vi "C2_controltower.vi"() -> ()   [LabVIEW 2012]
uses:
  <vilib>/LabVIEW Targets/FPGA/cRIO/cRIO-9505/controls.llb/_nicrio_cRIO-9505_DriveStatus.ctl
  <vilib>/FPGAPlugInAG/cRIO-9074/niLvFpga_Open_cRIO-9074.vi
  <vilib>/Utility/error.llb/Error Cluster From Error Code.vi
  <vilib>/rvi/errors/niLvFpgaAdjustHostInterfaceError.vi
  <vilib>/FPGAPlugInAG/cRIO-9074/niLvFpga_Close_cRIO-9074.vi
  <vilib>/rvi/interface/nirviOpenFPGA/nirviOpenFPGA.xnode
  FPGA Bitfiles/bbauvsbRIO_FPGATarget_FPGA9505Thruster_WhZwZzeic1g.lvbitx
  <vilib>/rvi/interface/nirviReadWriteControl/nirviReadWriteControl.xnode
  <vilib>/rvi/interface/nirviCloseFPGA/nirviCloseFPGA.xnode
  NiFpgaLv.dll
  <instrlib>/Ocean Server OS4000/Ocean Server OS4000.lvlib
panel:
  in  "Roll PID Gains":T1={"proportional gain (Kc)"=1.0, "integral time (Ti, min)"=0.01, "derivative time (Td, min)"=0.0}
  in  "Roll Setpoint":dbl
  out "Pwm Output":dbl
  out "Actual Roll":dbl
  out "Actual Heading":dbl
  in  "Baud Rate":u32(ring)=19200
  in  "Reset (True)":bool=TRUE
  in  "ID Query (False)":bool
  in  "Heading PID Gains":T1={"proportional gain (Kc)"=1.0, "integral time (Ti, min)"=0.01, "derivative time (Td, min)"=0.0}
  in  "Heading Setpoint":dbl
  out "Pwm Output":dbl
  in  "Manual Surge":dbl(slide)
  in  "Manual Yaw":dbl(slide)
  in  "Manual Depth":dbl(slide)
  in  "Manual Roll":dbl(slide)
  in  "Control Mode":T2(ring)
  in  "Depth PID Gains":T1={"proportional gain (Kc)"=1.0, "integral time (Ti, min)"=0.01, "derivative time (Td, min)"=0.0}
  in  "Depth Setpoint":dbl
  out "Pwm Output":dbl
  out "Actual Depth (m)":dbl(slide)
  in  "Atm Offset":dbl
  out "PSI":dbl(knob)
  out "Current Sense 2":i16
  out "Current Sense 1":i16
  out "Drive Status 1":T3
  out "Drive Status 2":T3
  in  "Enable 2":bool
  in  "Enable 1":bool
  in  "Disable 2":bool
  in  "Disable 1":bool
  in  "resource name":tag="RIO0::INSTR"
  out "error out":errorcluster
  in  "stop":bool
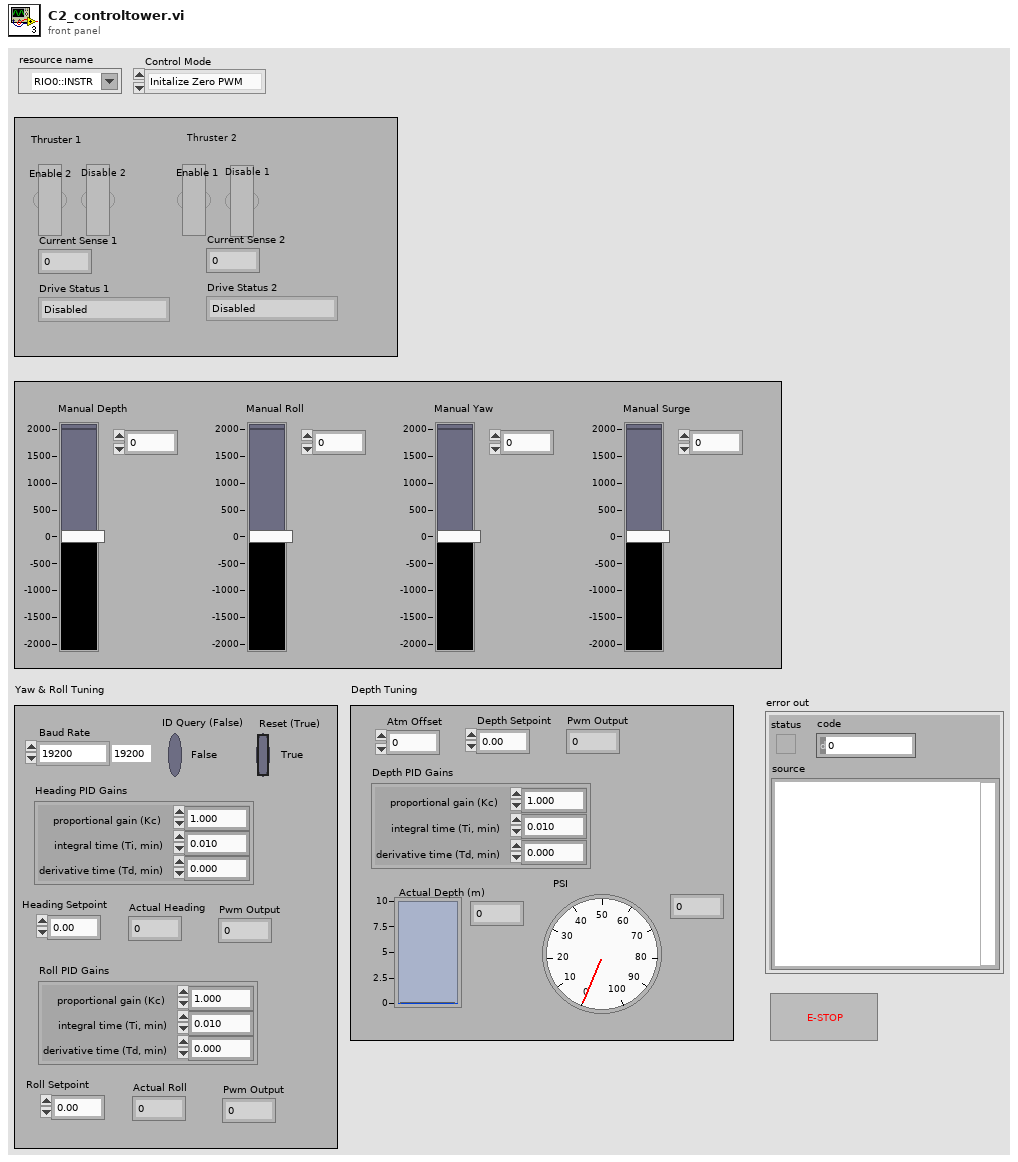
[diagram p1: front panel]
types:
  T1 = cluster{"proportional gain (Kc)":dbl, "integral time (Ti, min)":dbl, "derivative time (Td, min)":dbl}
  T2 = enum16{"Initalize Zero PWM", "Manual Depth", "Manual Roll", "Manual Yaw", "Manual Surge", "PID Depth", "PID Yaw", "PID Roll"}
  T3 = typedef "_nicrio_cRIO-9505_DriveStatus.ctl" = enum8{"Enabled", "Disabled", "Disabled by Drive Fault", "Disabled by Temp. Fault", "Disabled by E-Stop", "Unknown"}
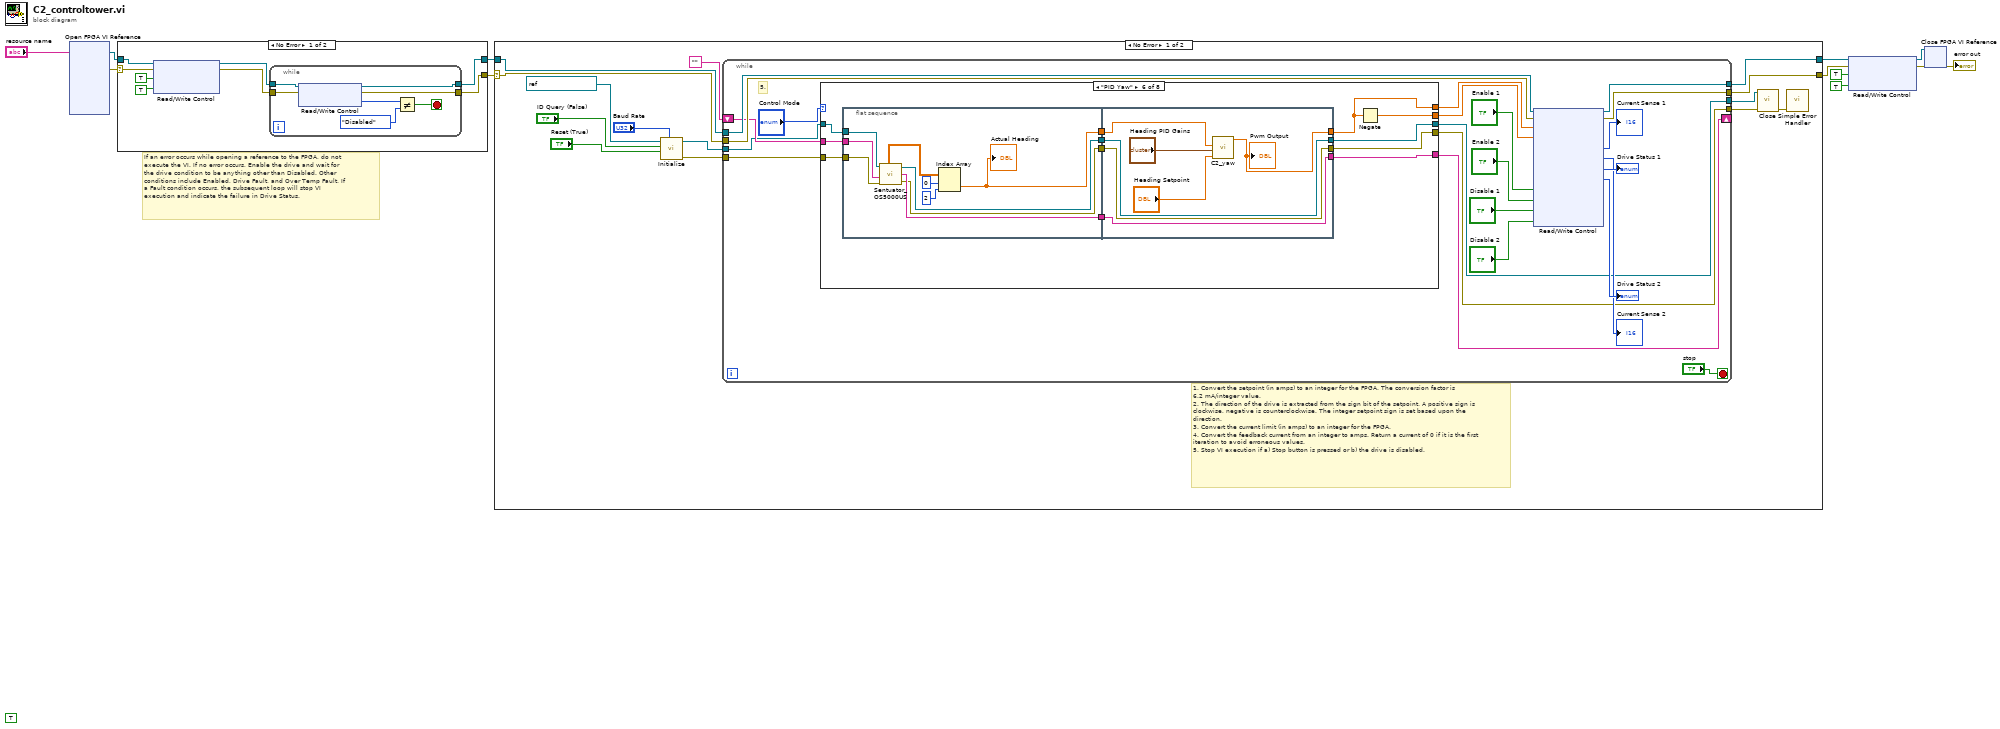
[diagram p0: block diagram]
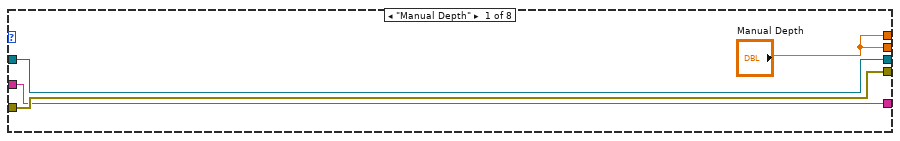
[diagram p2: hidden frame]
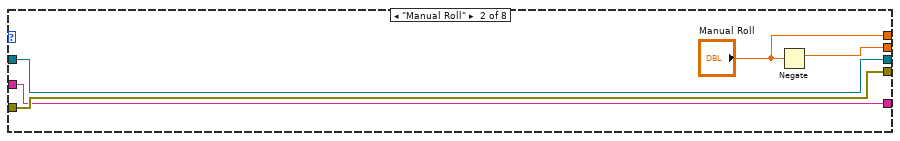
[diagram p3: hidden frame]
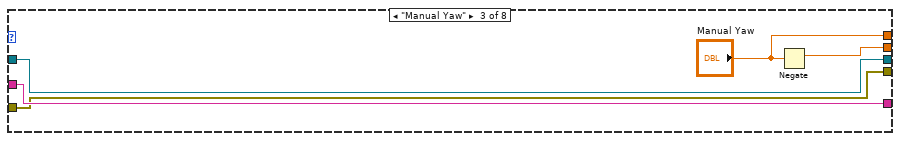
[diagram p4: hidden frame]
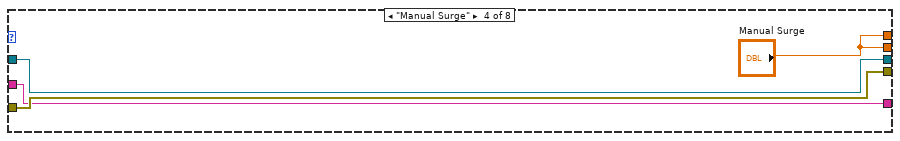
[diagram p5: hidden frame]
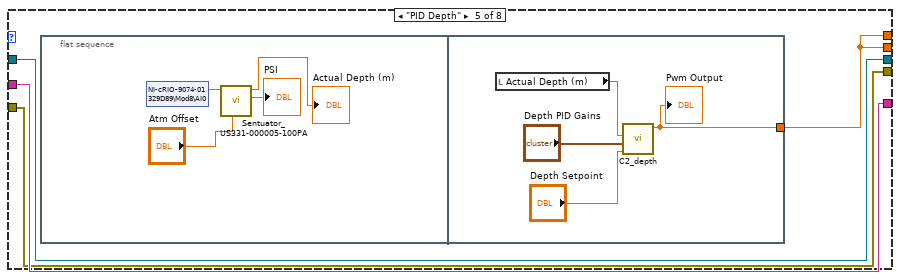
[diagram p6: hidden frame]
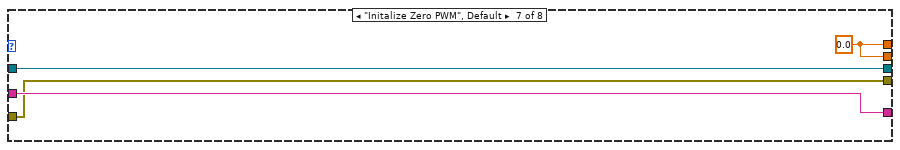
[diagram p7: hidden frame]
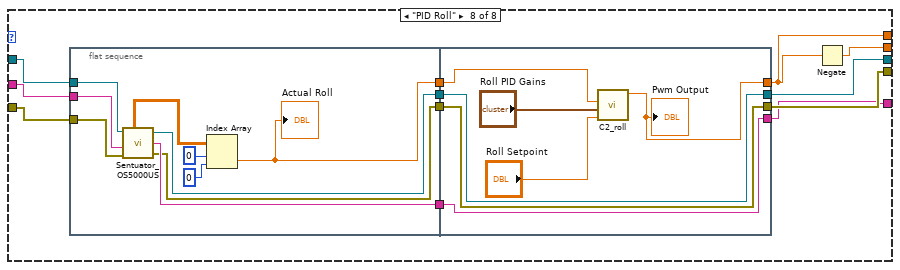
[diagram p8: hidden frame]
diagram:
  (unwired) TRUE
  # "If an error occurs while opening a reference to the FPGA, do not\nexecute the VI. If no error occurs, Enable the drive and wait for\nthe drive condition to be anything other than Disabled. Other\nconditions include Enabled, Drive Fault, and Over Temp Fault. If\na Fault condition occurs, the subsequent loop will stop VI\nexecution and indicate the failure in Drive Status."
  n1 = xnode "Open FPGA VI Reference"("resource name"="resource name") -> ("FPGA VI Reference Out"=w6:refnum<k20>, "error out"=w5:errorcluster)  [unwired: 1 in]
  n2 = case shown="No Error" w5 {
    selector: w5 -> [w15 w28]
    tunnel: w6 -> [w18 w29]
    tunnel: [w20 w29] -> w8
    tunnel: [w14 w28] -> w7
    frame No Error {
      n3 = xnode "Read/Write Control"("FPGA VI Reference In"=w18, "error in"=w15, "Enable Drive 1"=TRUE, "Enable Drive 2"=TRUE) -> ("FPGA VI Reference Out"=w17:refnum<k20>, "error out"=w16:errorcluster)
      n4 = while {
        tunnel: [w27] -> w20
        tunnel: w17 -> [w23]
        tunnel: w16 -> [w24]
        tunnel: [w21] -> w14
        stop <- w22 stop-if-true
        n5 = xnode "Read/Write Control"("FPGA VI Reference In"=w23, "error in"=w24) -> ("FPGA VI Reference Out"=w27:refnum<k20>, "error out"=w21:errorcluster, "Drive Status 1"=w26:T3)
        n6 = Not Equal?(x=w26, y=_nicrio_cRIO-9505_DriveStatus."Disabled") -> (x != y?=w22:bool)
      }
    }
    frame Error {
      # "Error occurred. Do not run."
    }
  }
  n7 = case shown="No Error" w7 {
    selector: w7 -> [w40 w158]
    tunnel: [w43 w159] -> w12
    tunnel: [w42 w158] -> w11
    tunnel: w8 -> [w41 w159]
    frame No Error {
      # "1. Convert the setpoint (in amps) to an integer for the FPGA. The conversion factor is \n6.2 mA/integer value.\n2. The direction of the drive is extracted from the sign bit of the setpoint. A positive sign is clockwise, negative is counterclockwise. The integer setpoint sign is set based upon the direction.\n3. Convert the current limit (in amps) to an integer for the FPGA.\n4. Convert the feedback current from an integer to amps. Return a current of 0 if it is the first iteration to avoid erroneous values.\n5. Stop VI execution if a) Stop button is pressed or b) the drive is disabled."
      n8 = call <instrlib>:"Initialize.vi"("Baud Rate"="Baud Rate", "Reset (True)"="Reset (True)", "ID Query (False)"="ID Query (False)", "VISA resource name"=refnum<visa-resource-name> refnum) -> ("error out"=w33:errorcluster, "VISA resource name out"=w34:refnum<visa-resource-name>)  [unwired: 6 in]
      n9 = while {
        tunnel: w41 -> [w65]
        tunnel: [w63] -> w43
        tunnel: w40 -> [w64]
        tunnel: [w62] -> w42
        tunnel: w34 -> [w50]
        tunnel: w33 -> [w49]
        shift-right: [w47] -> _
        shift-left: "" -> [w51]
        tunnel: [w48] -> w32
        tunnel: [w46] -> w31
        stop <- "stop" stop-if-true
        # "5."
        n10 = case shown="\"PID Yaw\"" "Control Mode" {
          tunnel: w51 -> [w66 w70 w76 w80 w85 w103 w126 w135]
          tunnel: w50 -> [w68 w72 w77 w82 w86 w102 w127 w136]
          tunnel: w49 -> [w67 w71 w75 w81 w84 w101 w125 w134]
          tunnel: [w68 w72 w77 w82 w86 w100 w127 w131] -> w48
          tunnel: [w66 w70 w76 w80 w85 w99 w126 w129] -> w47
          tunnel: [w67 w71 w75 w81 w84 w98 w125 w130] -> w46
          tunnel: ["Manual Depth" "Manual Roll" "Manual Yaw" "Manual Surge" w87 w96 w128 w133] -> w45
          tunnel: ["Manual Depth" w73 w78 "Manual Surge" w87 w97 w128 w132] -> w44
          frame "Manual Depth" {
          }
          frame "Manual Roll" {
            n11 = Negate(x="Manual Roll") -> (-x=w73:dbl)
          }
          frame "Manual Yaw" {
            n12 = Negate(x="Manual Yaw") -> (-x=w78:dbl)
          }
          frame "Manual Surge" {
          }
          frame "PID Depth" {
            n13 = flat-sequence {
              tunnel: [w92] -> w87
              frame #0 {
                n14 = shared-variable "NI-cRIO-9074-01329D89\\Mod8\\AI0"() -> (w90:dbl)  [unwired: 1 in, 1 out]
                n15 = call "Sentuator_US331-000005-100PA.vi"("Atm Offset"="Atm Offset", "Depth sensor \nVoltage"=w90) -> ("PSI"=→"PSI":dbl, "Actual Depth (m)"=→"Actual Depth (m)":dbl)  [unwired: 7 in, 1 out]
              }
              frame #1 {
                n16 = local read "Actual Depth (m)"() -> (w93:dbl)
                n17 = call "C2_depth.vi"("setpoint"="Depth Setpoint", "PID gains"="Depth PID Gains", "Actual Depth"=w93) -> ("Pwm Output"=w92:dbl)
                "Pwm Output" <- w92
              }
            }
          }
          frame "PID Yaw" {
            n18 = flat-sequence {
              tunnel: w103 -> [w117]
              tunnel: [w116] -> w107
              tunnel: [w115] -> w106
              tunnel: [w114] -> w105
              tunnel: [w108] -> w104
              tunnel: w102 -> [w110]
              tunnel: w101 -> [w109]
              tunnel: w107 -> [w124]
              tunnel: w106 -> [w123]
              tunnel: w105 -> [w119]
              tunnel: w104 -> [w120]
              tunnel: [w124] -> w100
              tunnel: [w123] -> w99
              tunnel: [w119] -> w98
              tunnel: [w118] -> w96
              frame #0 {
                n19 = call "Sentuator_OS5000US.vi"("VISA resource name"=w110, "Text to prepend to sentence"=w117, "error in (no error)"=w109) -> ("Angles"=w113:dbl[][], "VISA resource name out"=w116:refnum<visa-resource-name>, "Remaining Sentence"=w115:string, "error out"=w114:errorcluster)  [unwired: 1 in]
                n20 = Index Array(array=w113, index (row)=0, index (col)=2) -> (element=w108:dbl)
                "Actual Heading" <- w108
              }
              frame #1 {
                n21 = call "C2_yaw.vi"("setpoint"="Heading Setpoint", "PID gains"="Heading PID Gains", "Actual Heading"=w120) -> ("Pwm Output"=w118:dbl)
                "Pwm Output" <- w118
              }
            }
            n22 = Negate(x=w96) -> (-x=w97:dbl)
          }
          frame "Initalize Zero PWM", Default {
            w128 = 0.0
          }
          frame "PID Roll" {
            n23 = flat-sequence {
              tunnel: w135 -> [w150]
              tunnel: [w149] -> w140
              tunnel: [w148] -> w139
              tunnel: [w147] -> w138
              tunnel: [w141] -> w137
              tunnel: w136 -> [w143]
              tunnel: w134 -> [w142]
              tunnel: w140 -> [w157]
              tunnel: w139 -> [w156]
              tunnel: w138 -> [w152]
              tunnel: w137 -> [w153]
              tunnel: [w157] -> w131
              tunnel: [w156] -> w129
              tunnel: [w152] -> w130
              tunnel: [w151] -> w133
              frame #0 {
                n24 = call "Sentuator_OS5000US.vi"("VISA resource name"=w143, "Text to prepend to sentence"=w150, "error in (no error)"=w142) -> ("Angles"=w146:dbl[][], "VISA resource name out"=w149:refnum<visa-resource-name>, "Remaining Sentence"=w148:string, "error out"=w147:errorcluster)  [unwired: 1 in]
                n25 = Index Array(array=w146, index (row)=0, index (col)=0) -> (element=w141:dbl)
                "Actual Roll" <- w141
              }
              frame #1 {
                n26 = call "C2_roll.vi"("setpoint"="Roll Setpoint", "PID gains"="Roll PID Gains", "Actual Roll"=w153) -> ("Pwm Output"=w151:dbl)
                "Pwm Output" <- w151
              }
            }
            n27 = Negate(x=w133) -> (-x=w132:dbl)
          }
        }
        n28 = xnode "Read/Write Control"("FPGA VI Reference In"=w65, "error in"=w64, "Input PWM 1"=w45, "Input PWM 2"=w44, "Enable Drive 1"="Enable 1", "Enable Drive 2"="Enable 2", "Disable Drive 1"="Disable 1", "Disable Drive 2"="Disable 2") -> ("FPGA VI Reference Out"=w63:refnum<k20>, "error out"=w62:errorcluster, "Current Sense 1"=→"Current Sense 1":i16, "Current Sense 2"=→"Current Sense 2":i16, "Drive Status 1"=→"Drive Status 1":T3, "Drive Status 2"=→"Drive Status 2":T3)
      }
      n29 = call <instrlib>:"Close.vi"("error in (no error)"=w31, "VISA resource name"=w32) -> ("error out"=w36:errorcluster)  [unwired: 9 in]
      n30 = call <vilib>:"Simple Error Handler.vi"("error in (no error)"=w36) -> ()  [unwired: 1 in, 8 out]
    }
    frame Error {
      # "Error occurred. Do not run."
    }
  }
  n31 = xnode "Read/Write Control"("FPGA VI Reference In"=w12, "error in"=w11, "Disable Drive 1"=TRUE, "Disable Drive 2"=TRUE) -> ("FPGA VI Reference Out"=w10:refnum<k20>, "error out"=w9:errorcluster)
  n32 = xnode "Close FPGA VI Reference"("FPGA VI Reference In"=w10, "error in"=w9) -> ("error out"=→"error out":errorcluster)
